vi "decodeBoolean.vi"(8 "error in (no error)":errorcluster, 10 "ByteArray":u8[](array[numeric])) -> (0 "error out":errorcluster, 1 "Boolean":bool, 2 "variant":variant, 3 "RemainingBytes":u8[](array[numeric]), 5 "Type":string)   [LabVIEW 2020, in "MsgPack.lvlib"]
uses:
  MsgPack.lvlib
  <vilib>/Utility/error.llb/Error Cluster From Error Code.vi
  <vilib>/ErrorRing/Error Ring.xnode
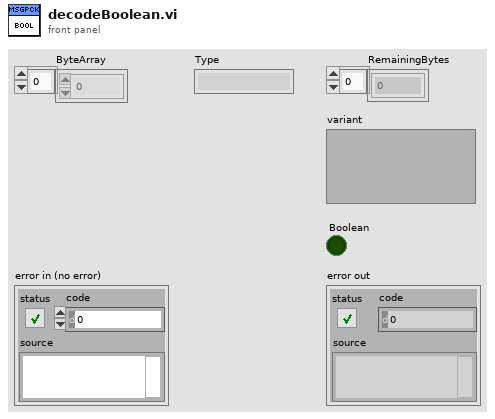
[diagram p1: front panel]
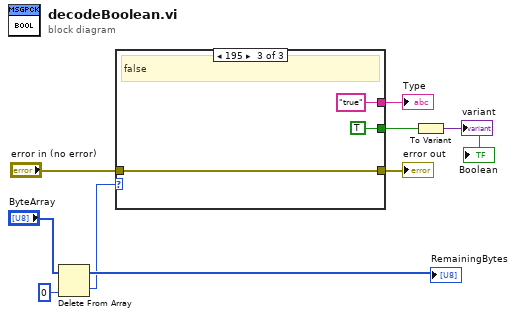
[diagram p0: block diagram]
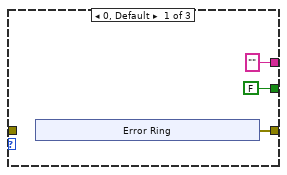
[diagram p2: hidden frame]
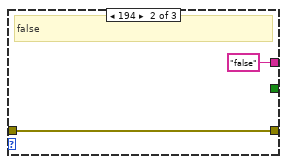
[diagram p3: hidden frame]
diagram:
  n1 = Delete From Array(array="ByteArray", index=0) -> (deleted portion=w1:u8, array with subset deleted=→"RemainingBytes":u8[])  [unwired: 1 in]
  n2 = case shown="195" w1 {
    tunnel: [w10 w19 w22] -> w8
    tunnel: "error in (no error)" -> [_ w19 w22]
    tunnel: ["" "false" "true"] -> w6
    tunnel: [FALSE _ TRUE] -> w5
    frame 0, Default {
      n3 = xnode "Error Ring"() -> ("error out"=w10:errorcluster)
    }
    frame 194 {
      # "false"
    }
    frame 195 {
      # "false"
    }
  }
  "error out" <- w8
  "Type" <- w6
  "Boolean" <- w5
  n4 = To Variant(anything=w5) -> (Variant=→"variant":variant)
